vi "OP4_FUNZIONAMENTO.vi"(0 "Esito 2 in":cluster{"Si":bool, "No":bool}, 1 "Esito 3 in":cluster{"Si":bool, "No":bool}, 2 "Esito 4 in":cluster{"Si":bool, "No":bool}, 3 "Esito 5 in":cluster{"Si":bool, "No":bool}, 4 "Esito 6 in":cluster{"Si":bool, "No":bool}, 5 "Esito 7 in":cluster{"Si":bool, "No":bool}, 6 "Esito 8 in":cluster{"Si":bool, "No":bool}, 7 "Esito 9 in":cluster{"Si":bool, "No":bool}, 8 "Esito 1 in":cluster{"Si":bool, "No":bool}, 9 "Tasto premuto":T2(array[ring]), 10 "Tipo specifica":string, 12 "Stato in":u16, 14 "Stato out":u16) -> (16 "Dato":string[](array[string]), 17 "ANNULLA PROVA":bool, 18 "Esito 1 out":T1, 19 "i out":i32=1, 20 "Esito 2 out":T1, 21 "Esito 3 out":T1, 22 "Esito 4 out":T1, 23 "Esito 5 out":T1, 24 "Esito 6 out":T1, 25 "Esito 7 out":T1, 26 "Esito 8 out":T1, 27 "Esito 9 out":T1)   [LabVIEW 2022 SP3]
uses:
  Labview/Globali.vi
panel:
  in  "i max":i32
  in  "i":i32=1
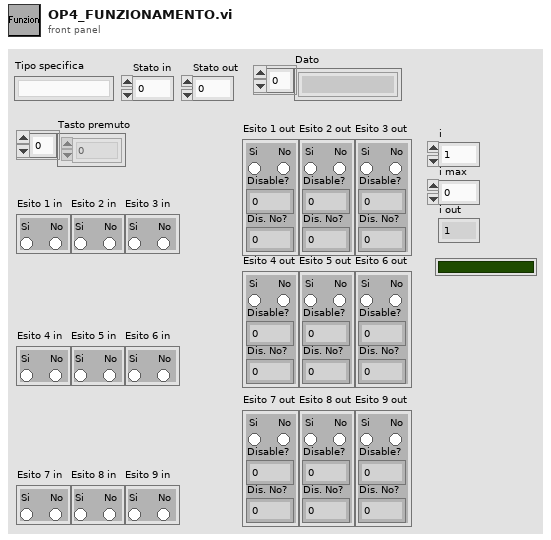
[diagram p1: front panel]
types:
  T1 = cluster{"Disable?":i16, "Si":bool, "No":bool, "Dis. No?":i16}
  T2 = enum16{"0", "1", "2", "3", "4", "5", "6", "7", "8", "9", "A", "B", "C", "D", "E", "F", "G", "H", "I", "J", "K", "L", "M", "N", "O", "P", "Q", "R", "S", "T", "U", "V", "W", "X", "Y", "Z", "F1", "F2", "F3", "F4", "F5", "F6", "F7", "F8", "F9", "F10", "F11", "F12", "F13", "F14", "F15", "ADD", "BACK", "BACKSLASH", "CAPITAL", "COMMA", "DECIMAL", "DELETE", "DIVIDE", "DOWN", "END", "EQUALS", "ESCAPE", "GRAVE (`)", "HOME", "INSERT", "LBRACKET", "LCONTROL", "LEFT", "L ALT", "LSHIFT", "LWIN", "MINUS", "MULTIPLY", "NEXT", "NUMLOCK", "NUMPAD_0", "NUMPAD_1", "NUMPAD_2", "NUMPAD_3", "NUMPAD_4", "NUMPAD_5", "NUMPAD_6", "NUMPAD_7", "NUMPAD_8", "NUMPAD_9", "PAUSE", "PERIOD", "PRIOR (PG UP)", "RBRACKET", "RCONTROL", "RETURN", "RIGHT", "R ALT", "RSHIFT", "RWIN", "SCROLL", "SEMICOLON", "SLASH", "SPACE", "SUBTRACT", "TAB", "UP", "ENTER (num pad)", "' (quote)"}[]
  T3 = cluster{"Dis. No?":i16, "No":bool, "Si":bool, "Disable?":i16}
  T4 = cluster{"Esito 1 out":cluster{"Disable?":i16, "Si":bool, "No":bool, "Dis. No?":i16}, "Esito 2 out":cluster{"Disable?":i16, "Si":bool, "No":bool, "Dis. No?":i16}, "Esito 3 out":cluster{"Disable?":i16, "Si":bool, "No":bool, "Dis. No?":i16}, "Esito 4 out":cluster{"Disable?":i16, "Si":bool, "No":bool, "Dis. No?":i16}, "Esito 5 out":cluster{"Disable?":i16, "Si":bool, "No":bool, "Dis. No?":i16}, "Esito 6 out":cluster{"Disable?":i16, "Si":bool, "No":bool, "Dis. No?":i16}, "Esito 7 out":cluster{"Disable?":i16, "Si":bool, "No":bool, "Dis. No?":i16}, "Esito 8 out":cluster{"Disable?":i16, "Si":bool, "No":bool, "Dis. No?":i16}, "Esito 9 out":cluster{"Disable?":i16, "Si":bool, "No":bool, "Dis. No?":i16}}
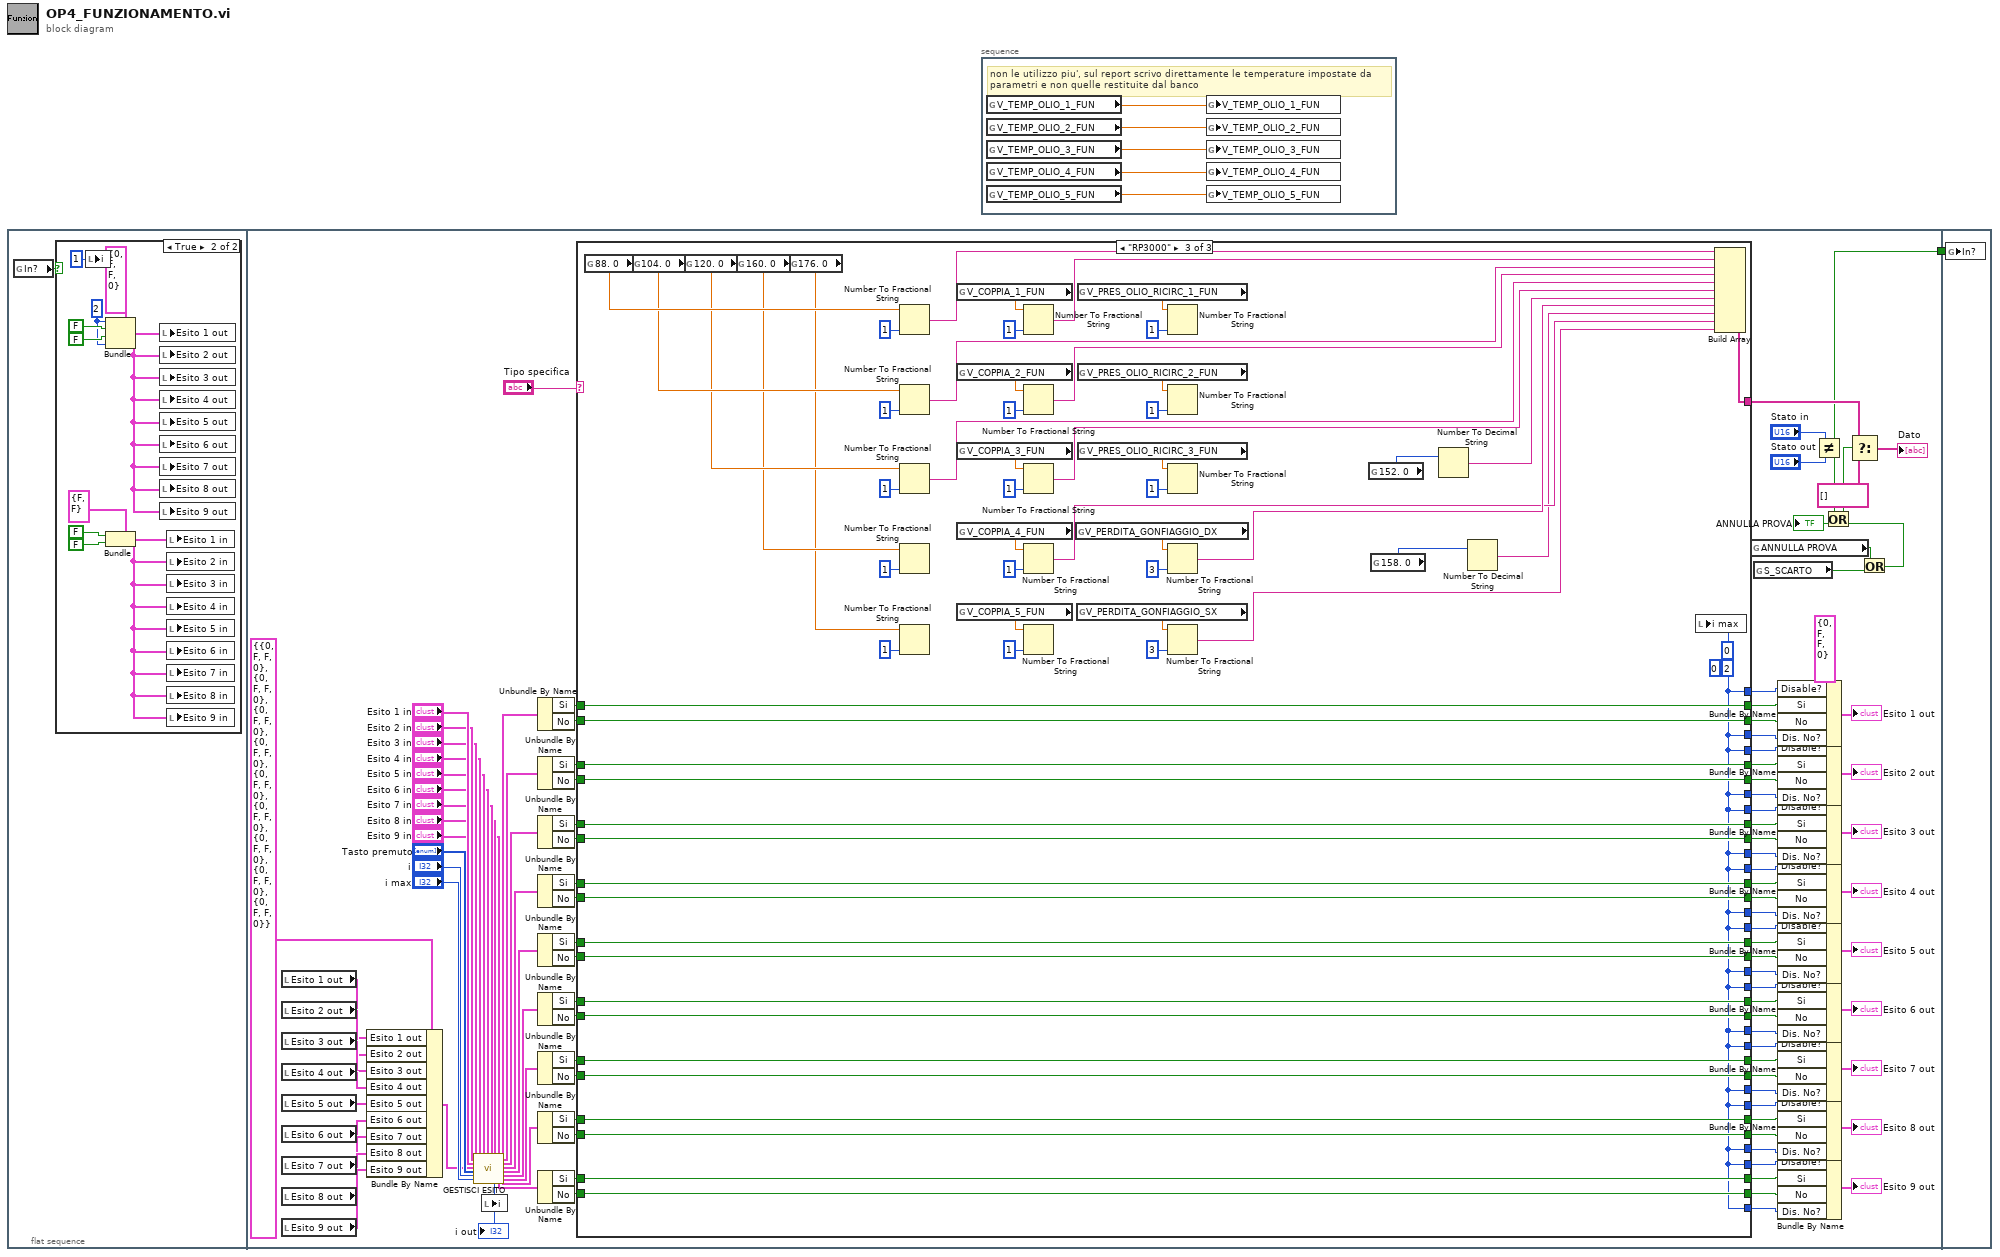
[diagram p0: block diagram]
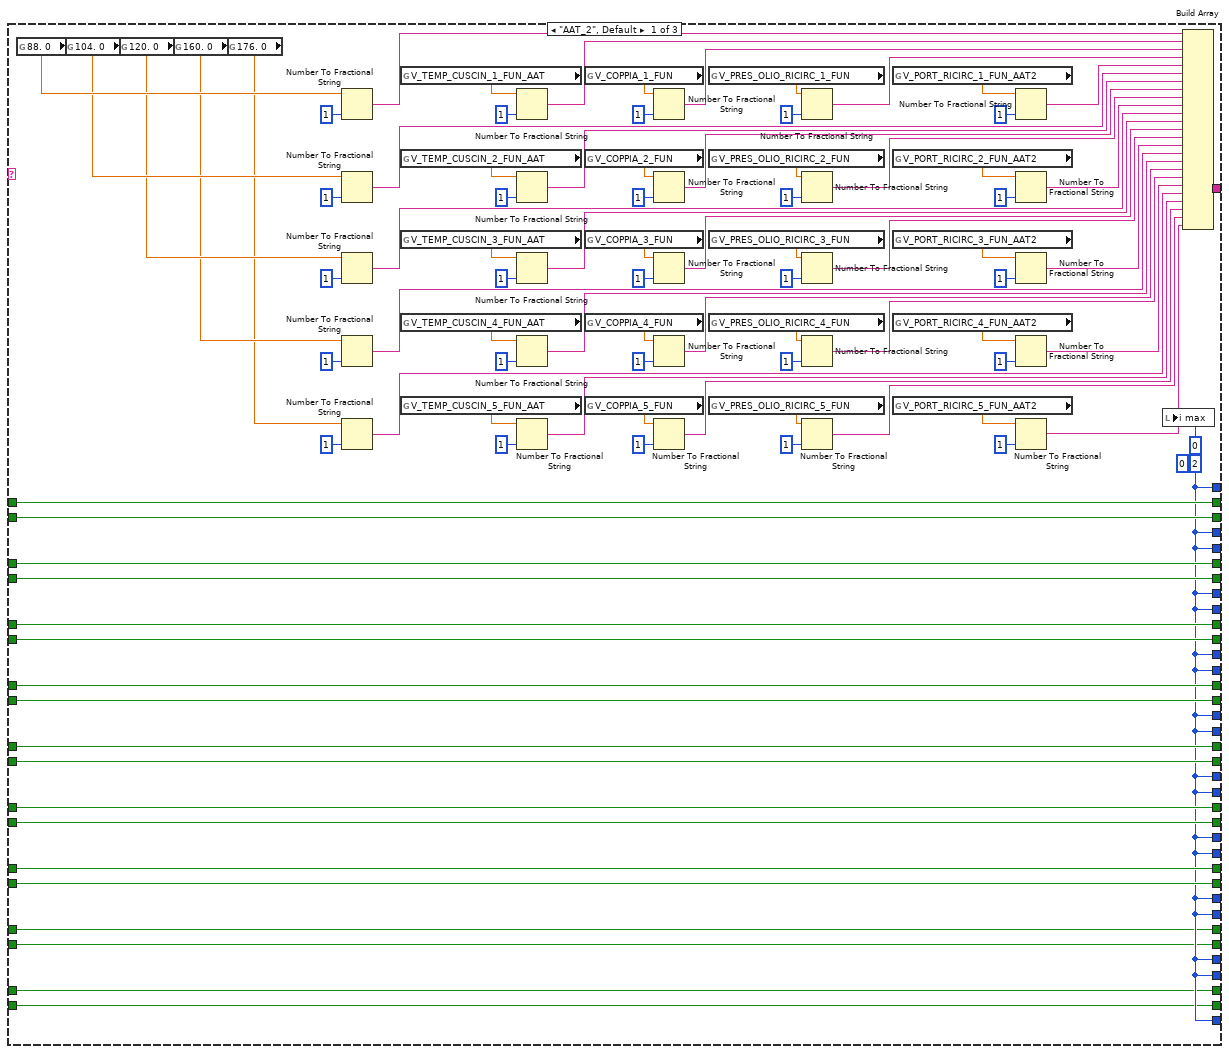
[diagram p3: hidden frame]
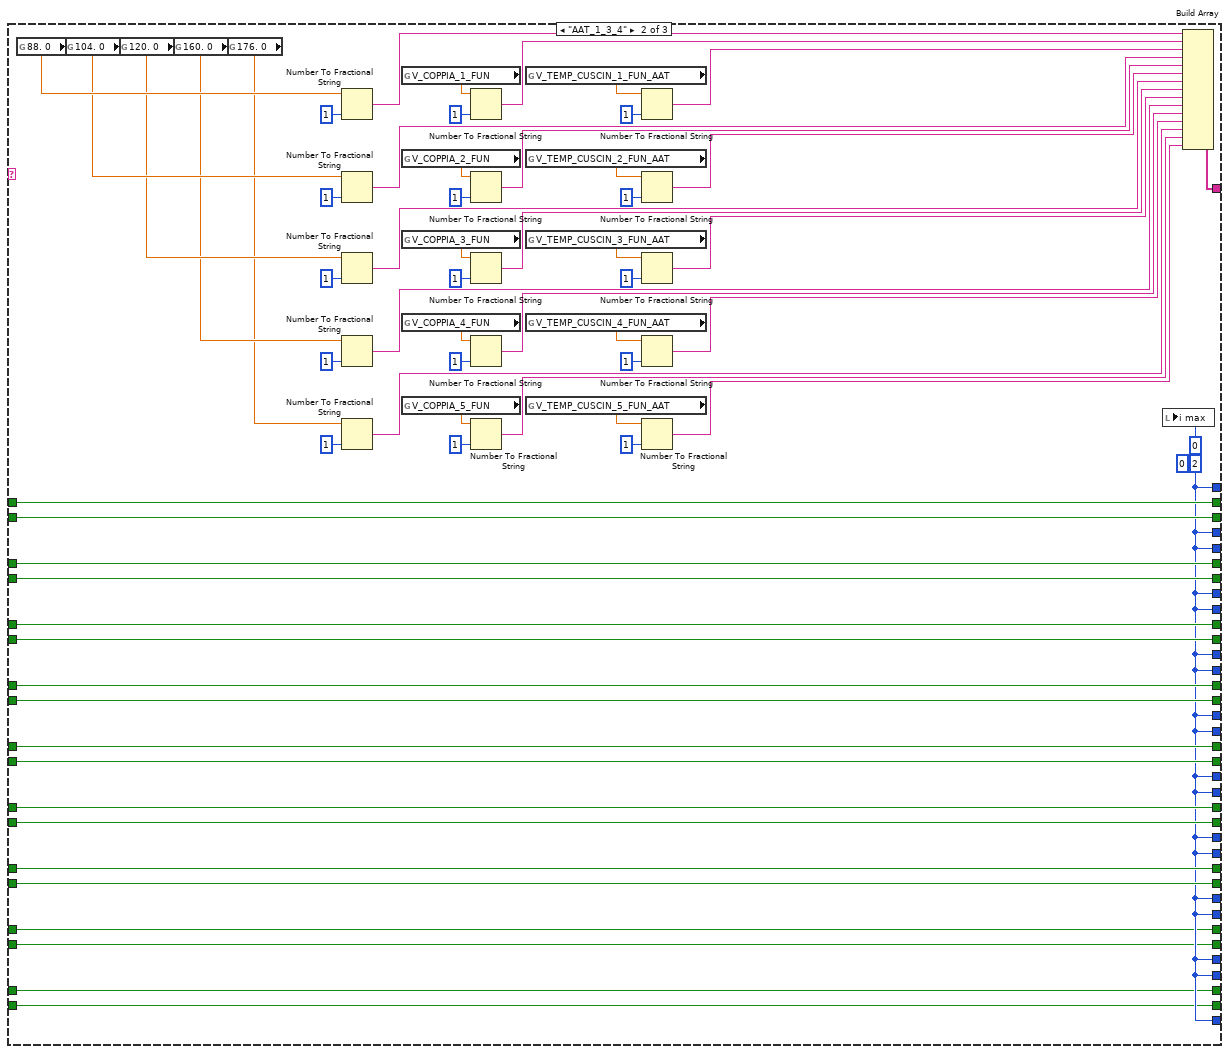
[diagram p4: hidden frame]
diagram:
  n1 = flat-sequence {
    tunnel: [w17] -> w1
    tunnel: w1 -> [w347]
    frame #0 {
      n2 = global read "Globali.vi" "In?"() -> (w2:bool)
      n3 = case shown="True" w2 {
        frame False {
        }
        frame True {
          w3 = i16 2 ("Disable?")
          n4 = local write "i"(1 ("i")) -> ()
          n5 = Bundle(cluster=T3 {"Dis. No?"=0, "No"=FALSE, "Si"=FALSE, "Disable?"=0} ("Esito 1 out"), "Dis. No?"=w3, "No"=FALSE ("Si"), "Si"=FALSE ("No"), "Disable?"=w3) -> (w5:T3)
          n6 = Bundle(cluster=cluster{"Si":bool, "No":bool} {"Si"=FALSE, "No"=FALSE} ("Esito 1 in"), "Si"=FALSE, "No"=FALSE) -> (w8:cluster{"Si":bool, "No":bool})
          n7 = local write "Esito 1 out"(w5) -> ()
          n8 = local write "Esito 2 out"(w5) -> ()
          n9 = local write "Esito 3 out"(w5) -> ()
          n10 = local write "Esito 4 out"(w5) -> ()
          n11 = local write "Esito 5 out"(w5) -> ()
          n12 = local write "Esito 6 out"(w5) -> ()
          n13 = local write "Esito 7 out"(w5) -> ()
          n14 = local write "Esito 8 out"(w5) -> ()
          n15 = local write "Esito 9 out"(w5) -> ()
          n16 = local write "Esito 1 in"(w8) -> ()
          n17 = local write "Esito 2 in"(w8) -> ()
          n18 = local write "Esito 3 in"(w8) -> ()
          n19 = local write "Esito 4 in"(w8) -> ()
          n20 = local write "Esito 5 in"(w8) -> ()
          n21 = local write "Esito 6 in"(w8) -> ()
          n22 = local write "Esito 7 in"(w8) -> ()
          n23 = local write "Esito 8 in"(w8) -> ()
          n24 = local write "Esito 9 in"(w8) -> ()
        }
      }
    }
    frame #1 {
      w68 = T1 {"Disable?"=0, "Si"=FALSE, "No"=FALSE, "Dis. No?"=0} ("Esito 1 out")
      n25 = local read "Esito 1 out"() -> (w84:T1)
      n26 = local read "Esito 2 out"() -> (w85:T1)
      n27 = local read "Esito 3 out"() -> (w86:T1)
      n28 = local read "Esito 4 out"() -> (w87:T1)
      n29 = local read "Esito 5 out"() -> (w88:T1)
      n30 = local read "Esito 6 out"() -> (w89:T1)
      n31 = local read "Esito 7 out"() -> (w90:T1)
      n32 = local read "Esito 8 out"() -> (w91:T1)
      n33 = local read "Esito 9 out"() -> (w92:T1)
      n34 = Bundle By Name(cluster=T4 {"Esito 1 out"={"Disable?"=0, "Si"=FALSE, "No"=FALSE, "Dis. No?"=0}, "Esito 2 out"={"Disable?"=0, "Si"=FALSE, "No"=FALSE, "Dis. No?"=0}, "Esito 3 out"={"Disable?"=0, "Si"=FALSE, "No"=FALSE, "Dis. No?"=0}, "Esito 4 out"={"Disable?"=0, "Si"=FALSE, "No"=FALSE, "Dis. No?"=0}, "Esito 5 out"={"Disable?"=0, "Si"=FALSE, "No"=FALSE, "Dis. No?"=0}, "Esito 6 out"={"Disable?"=0, "Si"=FALSE, "No"=FALSE, "Dis. No?"=0}, "Esito 7 out"={"Disable?"=0, "Si"=FALSE, "No"=FALSE, "Dis. No?"=0}, "Esito 8 out"={"Disable?"=0, "Si"=FALSE, "No"=FALSE, "Dis. No?"=0}, "Esito 9 out"={"Disable?"=0, "Si"=FALSE, "No"=FALSE, "Dis. No?"=0}} ("Cluster"), "Esito 1 out"=w84, "Esito 2 out"=w85, "Esito 3 out"=w86, "Esito 4 out"=w87, "Esito 5 out"=w88, "Esito 6 out"=w89, "Esito 7 out"=w90, "Esito 8 out"=w91, "Esito 9 out"=w92) -> (w93:T4)
      n35 = call "GESTISCI ESITO.vi"("Esito 3 in"="Esito 3 in", "Esito 2 in"="Esito 2 in", "Esito 1 in"="Esito 1 in", "Cluster"=w93, "Tasto premuto"="Tasto premuto", "i in"="i", "i max"="i max", "Esito 4 in"="Esito 4 in", "Esito 5 in"="Esito 5 in", "Esito 6 in"="Esito 6 in", "Esito 7 in"="Esito 7 in", "Esito 8 in"="Esito 8 in", "Esito 9 in"="Esito 9 in") -> ("i out"=w18:i32, "Esito 9 in 2"=w114:cluster{"Si":bool, "No":bool}, "Esito 1 in 2"=w106:cluster{"Si":bool, "No":bool}, "Esito 2 in 2"=w107:cluster{"Si":bool, "No":bool}, "Esito 3 in 2"=w108:cluster{"Si":bool, "No":bool}, "Esito 4 in 2"=w109:cluster{"Si":bool, "No":bool}, "Esito 5 in 2"=w110:cluster{"Si":bool, "No":bool}, "Esito 6 in 2"=w111:cluster{"Si":bool, "No":bool}, "Esito 7 in 2"=w112:cluster{"Si":bool, "No":bool}, "Esito 8 in 2"=w113:cluster{"Si":bool, "No":bool})  [unwired: 5 in]
      "i out" <- w18
      n36 = local write "i"(w18) -> ()
      n37 = Unbundle By Name(w106) -> ("Si"=w82:bool, "No"=w81:bool)
      n38 = Unbundle By Name(w107) -> ("Si"=w70:bool, "No"=w69:bool)
      n39 = Unbundle By Name(w108) -> ("Si"=w72:bool, "No"=w71:bool)
      n40 = Unbundle By Name(w109) -> ("Si"=w74:bool, "No"=w73:bool)
      n41 = Unbundle By Name(w110) -> ("Si"=w76:bool, "No"=w75:bool)
      n42 = Unbundle By Name(w111) -> ("Si"=w78:bool, "No"=w77:bool)
      n43 = Unbundle By Name(w112) -> ("Si"=w80:bool, "No"=w79:bool)
      n44 = Unbundle By Name(w113) -> ("Si"=w30:bool, "No"=w29:bool)
      n45 = Unbundle By Name(w114) -> ("Si"=w28:bool, "No"=w27:bool)
      n46 = case shown="\"RP3000\"" "Tipo specifica" {
        tunnel: [w146 w242 w313] -> w117
        tunnel: [w131 w226 w293] -> w58
        tunnel: [w131 w226 w293] -> w55
        tunnel: [w131 w226 w293] -> w46
        tunnel: [w131 w226 w293] -> w45
        tunnel: [w131 w226 w293] -> w44
        tunnel: [w131 w226 w293] -> w43
        tunnel: [w131 w226 w293] -> w42
        tunnel: [w131 w226 w293] -> w41
        tunnel: [w131 w226 w293] -> w40
        tunnel: [w145 w241 w312] -> w57
        tunnel: [w144 w240 w311] -> w56
        tunnel: [w132 w239 w294] -> w19
        tunnel: [w133 w238 w296] -> w25
        tunnel: [w134 w237 w297] -> w24
        tunnel: [w135 w236 w310] -> w26
        tunnel: [w136 w235 w309] -> w47
        tunnel: [w137 w234 w298] -> w23
        tunnel: [w138 w233 w299] -> w22
        tunnel: [w139 w232 w300] -> w21
        tunnel: [w140 w231 w301] -> w20
        tunnel: [w141 w230 w308] -> w48
        tunnel: [w142 w229 w307] -> w49
        tunnel: [w143 w228 w306] -> w50
        tunnel: [w127 w225 w303] -> w51
        tunnel: [w128 w224 w302] -> w52
        tunnel: [w130 w223 w305] -> w53
        tunnel: [w129 w222 w304] -> w54
        tunnel: w82 -> [w145 w241 w312]
        tunnel: w81 -> [w144 w240 w311]
        tunnel: w79 -> [w143 w228 w306]
        tunnel: w80 -> [w142 w229 w307]
        tunnel: w77 -> [w141 w230 w308]
        tunnel: w78 -> [w140 w231 w301]
        tunnel: w75 -> [w139 w232 w300]
        tunnel: w76 -> [w138 w233 w299]
        tunnel: w73 -> [w137 w234 w298]
        tunnel: w74 -> [w136 w235 w309]
        tunnel: w71 -> [w135 w236 w310]
        tunnel: w72 -> [w134 w237 w297]
        tunnel: w69 -> [w133 w238 w296]
        tunnel: w70 -> [w132 w239 w294]
        tunnel: [w131 w226 w293] -> w39
        tunnel: [w131 w226 w293] -> w38
        tunnel: [w131 w226 w293] -> w37
        tunnel: [w131 w226 w293] -> w36
        tunnel: [w131 w226 w293] -> w35
        tunnel: [w131 w226 w293] -> w34
        tunnel: [w131 w226 w293] -> w33
        tunnel: [w131 w226 w293] -> w32
        tunnel: [w131 w226 w293] -> w31
        tunnel: w30 -> [w127 w225 w303]
        tunnel: w29 -> [w128 w224 w302]
        tunnel: w28 -> [w130 w223 w305]
        tunnel: w27 -> [w129 w222 w304]
        frame "AAT_2", Default {
          w131 = i16 2
          (unwired) i16 0
          n47 = global read "Globali.vi" "88. 0"() -> (w125:sgl)
          n48 = global read "Globali.vi" "104. 0"() -> (w124:sgl)
          n49 = global read "Globali.vi" "120. 0"() -> (w123:sgl)
          n50 = global read "Globali.vi" "160. 0"() -> (w122:sgl)
          n51 = global read "Globali.vi" "176. 0"() -> (w121:sgl)
          n52 = Number To Fractional String(number=w125, precision (6)=i16 1) -> (F-format string=w147:string)  [unwired: 2 in]
          n53 = Number To Fractional String(number=w124, precision (6)=i16 1) -> (F-format string=w152:string)  [unwired: 2 in]
          n54 = Number To Fractional String(number=w123, precision (6)=i16 1) -> (F-format string=w167:string)  [unwired: 2 in]
          n55 = Number To Fractional String(number=w122, precision (6)=i16 1) -> (F-format string=w166:string)  [unwired: 2 in]
          n56 = Number To Fractional String(number=w121, precision (6)=i16 1) -> (F-format string=w161:string)  [unwired: 2 in]
          n57 = global read "Globali.vi" "V_TEMP_CUSCIN_1_FUN_AAT"() -> (w211:sgl)
          n58 = global read "Globali.vi" "V_TEMP_CUSCIN_2_FUN_AAT"() -> (w187:sgl)
          n59 = global read "Globali.vi" "V_TEMP_CUSCIN_3_FUN_AAT"() -> (w172:sgl)
          n60 = global read "Globali.vi" "V_TEMP_CUSCIN_4_FUN_AAT"() -> (w177:sgl)
          n61 = global read "Globali.vi" "V_TEMP_CUSCIN_5_FUN_AAT"() -> (w178:sgl)
          n62 = Number To Fractional String(number=w211, precision (6)=i16 1) -> (F-format string=w148:string)  [unwired: 2 in]
          n63 = Number To Fractional String(number=w187, precision (6)=i16 1) -> (F-format string=w153:string)  [unwired: 2 in]
          n64 = Number To Fractional String(number=w172, precision (6)=i16 1) -> (F-format string=w168:string)  [unwired: 2 in]
          n65 = Number To Fractional String(number=w177, precision (6)=i16 1) -> (F-format string=w165:string)  [unwired: 2 in]
          n66 = Number To Fractional String(number=w178, precision (6)=i16 1) -> (F-format string=w160:string)  [unwired: 2 in]
          n67 = global read "Globali.vi" "V_COPPIA_1_FUN"() -> (w210:sgl)
          n68 = global read "Globali.vi" "V_COPPIA_2_FUN"() -> (w186:sgl)
          n69 = global read "Globali.vi" "V_COPPIA_3_FUN"() -> (w173:sgl)
          n70 = global read "Globali.vi" "V_COPPIA_4_FUN"() -> (w176:sgl)
          n71 = global read "Globali.vi" "V_COPPIA_5_FUN"() -> (w179:sgl)
          n72 = Number To Fractional String(number=w210, precision (6)=i16 1) -> (F-format string=w149:string)  [unwired: 2 in]
          n73 = Number To Fractional String(number=w186, precision (6)=i16 1) -> (F-format string=w154:string)  [unwired: 2 in]
          n74 = Number To Fractional String(number=w173, precision (6)=i16 1) -> (F-format string=w171:string)  [unwired: 2 in]
          n75 = Number To Fractional String(number=w176, precision (6)=i16 1) -> (F-format string=w164:string)  [unwired: 2 in]
          n76 = Number To Fractional String(number=w179, precision (6)=i16 1) -> (F-format string=w159:string)  [unwired: 2 in]
          n77 = global read "Globali.vi" "V_PRES_OLIO_RICIRC_1_FUN"() -> (w209:sgl)
          n78 = global read "Globali.vi" "V_PRES_OLIO_RICIRC_2_FUN"() -> (w185:sgl)
          n79 = global read "Globali.vi" "V_PRES_OLIO_RICIRC_3_FUN"() -> (w174:sgl)
          n80 = global read "Globali.vi" "V_PRES_OLIO_RICIRC_4_FUN"() -> (w175:sgl)
          n81 = global read "Globali.vi" "V_PRES_OLIO_RICIRC_5_FUN"() -> (w180:sgl)
          n82 = Number To Fractional String(number=w209, precision (6)=i16 1) -> (F-format string=w150:string)  [unwired: 2 in]
          n83 = Number To Fractional String(number=w185, precision (6)=i16 1) -> (F-format string=w155:string)  [unwired: 2 in]
          n84 = Number To Fractional String(number=w174, precision (6)=i16 1) -> (F-format string=w170:string)  [unwired: 2 in]
          n85 = Number To Fractional String(number=w175, precision (6)=i16 1) -> (F-format string=w163:string)  [unwired: 2 in]
          n86 = Number To Fractional String(number=w180, precision (6)=i16 1) -> (F-format string=w158:string)  [unwired: 2 in]
          n87 = global read "Globali.vi" "V_PORT_RICIRC_1_FUN_AAT2"() -> (w208:sgl)
          n88 = global read "Globali.vi" "V_PORT_RICIRC_2_FUN_AAT2"() -> (w184:sgl)
          n89 = global read "Globali.vi" "V_PORT_RICIRC_3_FUN_AAT2"() -> (w183:sgl)
          n90 = global read "Globali.vi" "V_PORT_RICIRC_4_FUN_AAT2"() -> (w182:sgl)
          n91 = global read "Globali.vi" "V_PORT_RICIRC_5_FUN_AAT2"() -> (w181:sgl)
          n92 = Number To Fractional String(number=w208, precision (6)=i16 1) -> (F-format string=w151:string)  [unwired: 2 in]
          n93 = Number To Fractional String(number=w184, precision (6)=i16 1) -> (F-format string=w156:string)  [unwired: 2 in]
          n94 = Number To Fractional String(number=w183, precision (6)=i16 1) -> (F-format string=w169:string)  [unwired: 2 in]
          n95 = Number To Fractional String(number=w182, precision (6)=i16 1) -> (F-format string=w162:string)  [unwired: 2 in]
          n96 = Number To Fractional String(number=w181, precision (6)=i16 1) -> (F-format string=w157:string)  [unwired: 2 in]
          n97 = local write "i max"(0) -> ()
          n98 = Build Array(w147, w148, w149, w150, w151, w152, w153, w154, w155, w156, w167, w168, w171, w170, w169, w166, w165, w164, w163, w162, w161, w160, w159, w158, w157) -> (w146:string[])
        }
        frame "AAT_1_3_4" {
          w226 = 2
          (unwired) 0
          n99 = global read "Globali.vi" "88. 0"() -> (w221:sgl)
          n100 = global read "Globali.vi" "104. 0"() -> (w220:sgl)
          n101 = global read "Globali.vi" "120. 0"() -> (w219:sgl)
          n102 = global read "Globali.vi" "160. 0"() -> (w218:sgl)
          n103 = global read "Globali.vi" "176. 0"() -> (w217:sgl)
          n104 = Number To Fractional String(number=w221, precision (6)=i16 1) -> (F-format string=w243:string)  [unwired: 2 in]
          n105 = Number To Fractional String(number=w220, precision (6)=i16 1) -> (F-format string=w244:string)  [unwired: 2 in]
          n106 = Number To Fractional String(number=w219, precision (6)=i16 1) -> (F-format string=w247:string)  [unwired: 2 in]
          n107 = Number To Fractional String(number=w218, precision (6)=i16 1) -> (F-format string=w246:string)  [unwired: 2 in]
          n108 = Number To Fractional String(number=w217, precision (6)=i16 1) -> (F-format string=w245:string)  [unwired: 2 in]
          n109 = global read "Globali.vi" "V_COPPIA_1_FUN"() -> (w268:sgl)
          n110 = global read "Globali.vi" "V_COPPIA_2_FUN"() -> (w254:sgl)
          n111 = global read "Globali.vi" "V_COPPIA_3_FUN"() -> (w249:sgl)
          n112 = global read "Globali.vi" "V_COPPIA_4_FUN"() -> (w250:sgl)
          n113 = global read "Globali.vi" "V_COPPIA_5_FUN"() -> (w253:sgl)
          n114 = Number To Fractional String(number=w268, precision (6)=i16 1) -> (F-format string=w273:string)  [unwired: 2 in]
          n115 = Number To Fractional String(number=w254, precision (6)=i16 1) -> (F-format string=w275:string)  [unwired: 2 in]
          n116 = Number To Fractional String(number=w249, precision (6)=i16 1) -> (F-format string=w277:string)  [unwired: 2 in]
          n117 = Number To Fractional String(number=w250, precision (6)=i16 1) -> (F-format string=w279:string)  [unwired: 2 in]
          n118 = Number To Fractional String(number=w253, precision (6)=i16 1) -> (F-format string=w281:string)  [unwired: 2 in]
          n119 = global read "Globali.vi" "V_TEMP_CUSCIN_1_FUN_AAT"() -> (w269:sgl)
          n120 = global read "Globali.vi" "V_TEMP_CUSCIN_2_FUN_AAT"() -> (w255:sgl)
          n121 = global read "Globali.vi" "V_TEMP_CUSCIN_3_FUN_AAT"() -> (w248:sgl)
          n122 = global read "Globali.vi" "V_TEMP_CUSCIN_4_FUN_AAT"() -> (w251:sgl)
          n123 = global read "Globali.vi" "V_TEMP_CUSCIN_5_FUN_AAT"() -> (w252:sgl)
          n124 = Number To Fractional String(number=w269, precision (6)=i16 1) -> (F-format string=w274:string)  [unwired: 2 in]
          n125 = Number To Fractional String(number=w255, precision (6)=i16 1) -> (F-format string=w276:string)  [unwired: 2 in]
          n126 = Number To Fractional String(number=w248, precision (6)=i16 1) -> (F-format string=w278:string)  [unwired: 2 in]
          n127 = Number To Fractional String(number=w251, precision (6)=i16 1) -> (F-format string=w280:string)  [unwired: 2 in]
          n128 = Number To Fractional String(number=w252, precision (6)=i16 1) -> (F-format string=w282:string)  [unwired: 2 in]
          n129 = local write "i max"(0) -> ()
          n130 = Build Array(w243, w273, w274, w244, w275, w276, w247, w277, w278, w246, w279, w280, w245, w281, w282) -> (w242:string[])
        }
        frame "RP3000" {
          w293 = 2
          (unwired) 0
          n131 = global read "Globali.vi" "88. 0"() -> (w287:sgl)
          n132 = global read "Globali.vi" "104. 0"() -> (w286:sgl)
          n133 = global read "Globali.vi" "120. 0"() -> (w285:sgl)
          n134 = global read "Globali.vi" "160. 0"() -> (w284:sgl)
          n135 = global read "Globali.vi" "176. 0"() -> (w283:sgl)
          n136 = Number To Fractional String(number=w287, precision (6)=i16 1) -> (F-format string=w314:string)  [unwired: 2 in]
          n137 = Number To Fractional String(number=w286, precision (6)=i16 1) -> (F-format string=w316:string)  [unwired: 2 in]
          n138 = Number To Fractional String(number=w285, precision (6)=i16 1) -> (F-format string=w320:string)  [unwired: 2 in]
          n139 = Number To Fractional String(number=w284, precision (6)=i16 1) -> ()  [unwired: 2 in, 1 out]
          n140 = Number To Fractional String(number=w283, precision (6)=i16 1) -> ()  [unwired: 2 in, 1 out]
          n141 = global read "Globali.vi" "V_COPPIA_1_FUN"() -> (w343:sgl)
          n142 = global read "Globali.vi" "V_COPPIA_2_FUN"() -> (w329:sgl)
          n143 = global read "Globali.vi" "V_COPPIA_3_FUN"() -> (w322:sgl)
          n144 = global read "Globali.vi" "V_COPPIA_4_FUN"() -> (w325:sgl)
          n145 = global read "Globali.vi" "V_COPPIA_5_FUN"() -> (w326:sgl)
          n146 = Number To Fractional String(number=w343, precision (6)=i16 1) -> (F-format string=w315:string)  [unwired: 2 in]
          n147 = Number To Fractional String(number=w329, precision (6)=i16 1) -> (F-format string=w317:string)  [unwired: 2 in]
          n148 = Number To Fractional String(number=w322, precision (6)=i16 1) -> (F-format string=w321:string)  [unwired: 2 in]
          n149 = Number To Fractional String(number=w325, precision (6)=i16 1) -> (F-format string=w292:string)  [unwired: 2 in]
          n150 = Number To Fractional String(number=w326, precision (6)=i16 1) -> ()  [unwired: 2 in, 1 out]
          n151 = global read "Globali.vi" "V_PERDITA_GONFIAGGIO_DX"() -> (w324:sgl)
          n152 = global read "Globali.vi" "V_PERDITA_GONFIAGGIO_SX"() -> (w327:sgl)
          n153 = global read "Globali.vi" "V_PRES_OLIO_RICIRC_1_FUN"() -> (w342:sgl)
          n154 = global read "Globali.vi" "V_PRES_OLIO_RICIRC_2_FUN"() -> (w328:sgl)
          n155 = global read "Globali.vi" "V_PRES_OLIO_RICIRC_3_FUN"() -> (w323:sgl)
          n156 = Number To Fractional String(number=w342, precision (6)=i16 1) -> ()  [unwired: 2 in, 1 out]
          n157 = Number To Fractional String(number=w328, precision (6)=i16 1) -> ()  [unwired: 2 in, 1 out]
          n158 = Number To Fractional String(number=w323, precision (6)=i16 1) -> ()  [unwired: 2 in, 1 out]
          n159 = Number To Fractional String(number=w324, precision (6)=i16 3) -> (F-format string=w319:string)  [unwired: 2 in]
          n160 = Number To Fractional String(number=w327, precision (6)=i16 3) -> (F-format string=w318:string)  [unwired: 2 in]
          n161 = global read "Globali.vi" "152. 0"() -> (w290:u16)
          n162 = global read "Globali.vi" "158. 0"() -> (w289:u16)
          n163 = Number To Decimal String(number=w290) -> (decimal integer string=w291:string)  [unwired: 1 in]
          n164 = Number To Decimal String(number=w289) -> (decimal integer string=w288:string)  [unwired: 1 in]
          n165 = local write "i max"(0) -> ()
          n166 = Build Array(w314, w315, w316, w317, w320, w321, w291, w319, w288, w292, w318) -> (w313:string[])
        }
      }
      n167 = global read "Globali.vi" "ANNULLA PROVA"() -> (w15:bool)
      n168 = global read "Globali.vi" "S_SCARTO"() -> (w14:bool)
      n169 = Bundle By Name(cluster=w68, "Disable?"=w58, "Si"=w57, "No"=w56, "Dis. No?"=w31) -> (→"Esito 1 out":T1)
      n170 = Bundle By Name(cluster=w68, "Disable?"=w55, "Si"=w19, "No"=w25, "Dis. No?"=w32) -> (→"Esito 2 out":T1)
      n171 = Bundle By Name(cluster=w68, "Disable?"=w46, "Si"=w24, "No"=w26, "Dis. No?"=w33) -> (→"Esito 3 out":T1)
      n172 = Bundle By Name(cluster=w68, "Disable?"=w45, "Si"=w47, "No"=w23, "Dis. No?"=w34) -> (→"Esito 4 out":T1)
      n173 = Bundle By Name(cluster=w68, "Disable?"=w44, "Si"=w22, "No"=w21, "Dis. No?"=w35) -> (→"Esito 5 out":T1)
      n174 = Bundle By Name(cluster=w68, "Disable?"=w43, "Si"=w20, "No"=w48, "Dis. No?"=w36) -> (→"Esito 6 out":T1)
      n175 = Bundle By Name(cluster=w68, "Disable?"=w42, "Si"=w49, "No"=w50, "Dis. No?"=w37) -> (→"Esito 7 out":T1)
      n176 = Bundle By Name(cluster=w68, "Disable?"=w41, "Si"=w51, "No"=w52, "Dis. No?"=w38) -> (→"Esito 8 out":T1)
      n177 = Bundle By Name(cluster=w68, "Disable?"=w40, "Si"=w53, "No"=w54, "Dis. No?"=w39) -> (→"Esito 9 out":T1)
      n178 = Not Equal?(x="Stato in", y="Stato out") -> (x != y?=w17:bool)
      n179 = Or(x=w15, y=w14) -> (x .or. y?=w13:bool)
      "ANNULLA PROVA" <- w13
      n180 = Or(x=w17, y=w13) -> (x .or. y?=w16:bool)
      n181 = Select(t=w117, s=w16, f=string[] [] ("Dato")) -> (s? t:f=→"Dato":string[])
    }
    frame #2 {
      n182 = global write "Globali.vi" "In?"(w347) -> ()
    }
  }
  n183 = stacked-sequence {
    frame #0 {
      # "non le utilizzo piu', sul report scrivo direttamente le temperature impostate da \nparametri e non quelle restituite dal banco"
      n184 = global read "Globali.vi" "V_TEMP_OLIO_1_FUN"() -> (w352:sgl)
      n185 = global read "Globali.vi" "V_TEMP_OLIO_2_FUN"() -> (w351:sgl)
      n186 = global read "Globali.vi" "V_TEMP_OLIO_3_FUN"() -> (w350:sgl)
      n187 = global read "Globali.vi" "V_TEMP_OLIO_4_FUN"() -> (w349:sgl)
      n188 = global read "Globali.vi" "V_TEMP_OLIO_5_FUN"() -> (w348:sgl)
      n189 = global write "Globali.vi" "V_TEMP_OLIO_1_FUN"(w352) -> ()
      n190 = global write "Globali.vi" "V_TEMP_OLIO_2_FUN"(w351) -> ()
      n191 = global write "Globali.vi" "V_TEMP_OLIO_3_FUN"(w350) -> ()
      n192 = global write "Globali.vi" "V_TEMP_OLIO_4_FUN"(w349) -> ()
      n193 = global write "Globali.vi" "V_TEMP_OLIO_5_FUN"(w348) -> ()
    }
  }
